vi "Display Tools.vi"(5 "All Default Shortcuts":string[](array[string]), 7 "All Possible Shortcuts":string[](array[string]), 8 "Error In":errorcluster, 10 "Tools":refnum<class "Tools.lvclass">[](array[class]), 11 "Tools Tree Control":refnum<vi>) -> (0 "Error Out":errorcluster, 3 "Shortcuts":map{string, string}(c390))   [LabVIEW 2021, in "Seq Edit Quick Drop.lvlib"]
uses:
  Seq Edit Quick Drop.lvlib
  Dependencies/Tool Menu Utility.lvlibp/Tools/Tools.lvclass
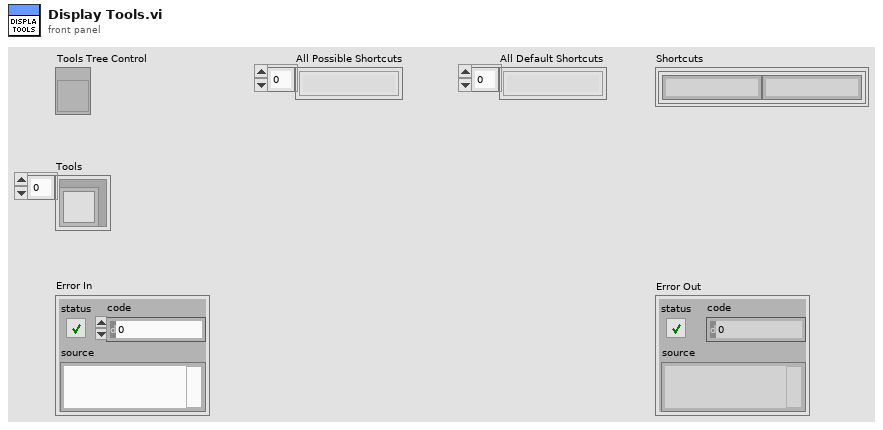
[diagram p1: front panel]
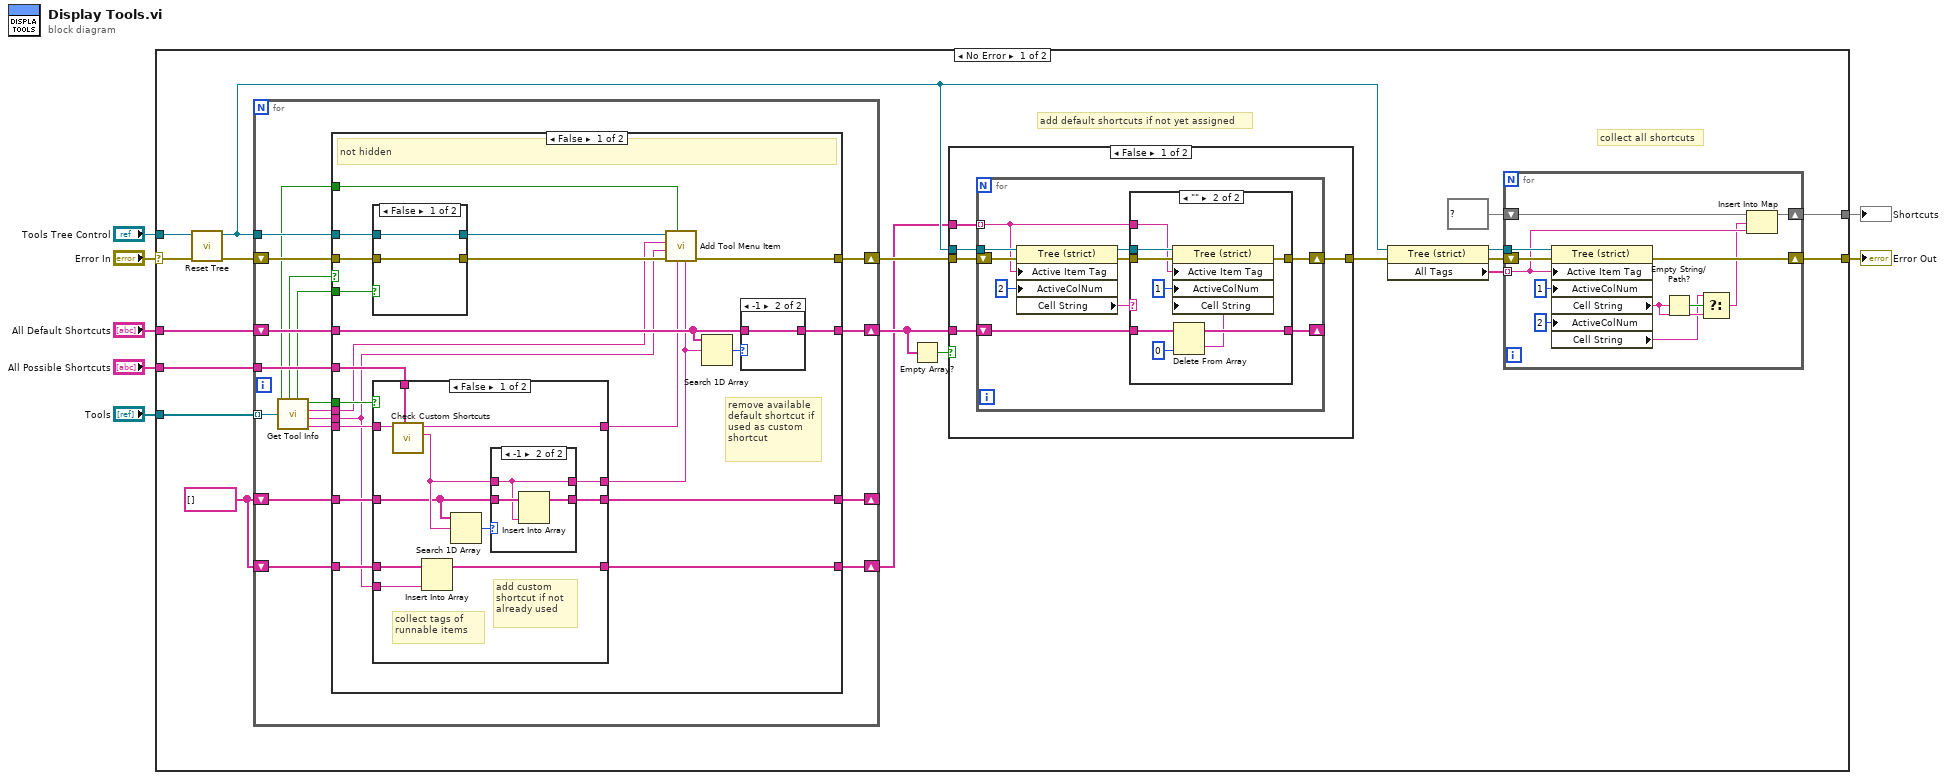
[diagram p0: block diagram]
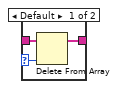
[diagram p4: hidden frame]
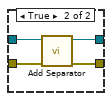
[diagram p5: hidden frame]
diagram:
  n1 = case shown="No Error" "Error In" {
    selector: "Error In" -> [w24 w137]
    tunnel: "Tools" -> [w22 _]
    tunnel: "Tools Tree Control" -> [w25 _]
    tunnel: [w8 w137] -> w4
    tunnel: "All Possible Shortcuts" -> [w23 _]
    tunnel: "All Default Shortcuts" -> [w20 _]
    tunnel: [w13 _] -> w3
    frame No Error {
      w12 = string[] []
      # "collect all shortcuts"
      # "add default shortcuts if not yet assigned"
      n2 = call "Reset Tree.vi"("error in (no error)"=w24, "TreeControl in"=w25) -> ("error out"=w26:errorcluster, "TreeControl out"=w17:refnum<vi>)  [unwired: 8 in]
      n3 = for {
        tunnel: w17 -> [w82]
        shift-right: [w75] -> w21
        shift-left: w26 -> [w83]
        tunnel: w22 -> [w72] mode=indexing
        tunnel: w23 -> [w81]
        shift-right: [w71] -> w19
        shift-left: w20 -> [w80]
        shift-right: [w69] -> _
        shift-left: w12 -> [w70]
        shift-right: [w67] -> w11
        shift-left: w12 -> [w68]
        n4 = call "Get Tool Info.vi"("Tool"=w72) -> ("Enabled?"=w66:bool, "Hidden?"=w74:bool, "Separator Before?"=w73:bool, "Submenu?"=w79:bool, "Parent ID"=w78:string, "ID"=w76:string, "Item Text"=w77:string)  [unwired: 3 in]
        n5 = case shown="False" w74 {
          tunnel: w83 -> [w100 w136]
          tunnel: w82 -> [w99 _]
          tunnel: [w98 w136] -> w75
          tunnel: w73 -> [w97 _]
          tunnel: w79 -> [w95 _]
          tunnel: w78 -> [w89 _]
          tunnel: w77 -> [w96 _]
          tunnel: w76 -> [w84 _]
          tunnel: w81 -> [w92 _]
          tunnel: w80 -> [w102 w135]
          tunnel: [w93 w135] -> w71
          tunnel: w70 -> [w104 w134]
          tunnel: [w103 w134] -> w69
          tunnel: w66 -> [w90 _]
          tunnel: w68 -> [w86 w133]
          tunnel: [w85 w133] -> w67
          frame False {
            # "remove available default shortcut if used as custom shortcut"
            # "not hidden"
            n6 = case shown="False" w97 {
              tunnel: w100 -> [w109 w114]
              tunnel: w99 -> [w110 w113]
              tunnel: [w110 w111] -> w91
              tunnel: [w109 w112] -> w101
              frame False {
              }
              frame True {
                n7 = call "Add Separator.vi"("error in (no error)"=w114, "TreeControl in"=w113) -> ("error out"=w112:errorcluster, "TreeControl out"=w111:refnum<vi>)  [unwired: 8 in]
              }
            }
            n8 = case shown="False" w95 {
              tunnel: w92 -> [w125 _]
              tunnel: w96 -> [w124 w132]
              tunnel: [w123 w132] -> w87
              tunnel: [w121 _] -> w88
              tunnel: w104 -> [w118 w131]
              tunnel: [w120 w131] -> w103
              tunnel: w86 -> [w117 w130]
              tunnel: [w116 w130] -> w85
              tunnel: w84 -> [w115 _]
              frame False {
                # "add custom shortcut if not already used"
                # "collect tags of runnable items"
                n9 = call "Check Custom Shortcuts.vi"("All Possible Shortcuts"=w125, "Item Text"=w124) -> ("Shortcut"=w119:string, "Name"=w123:string)  [unwired: 8 in]
                n10 = Insert Into Array(array=w117, new element=w115) -> (w116:string[])  [unwired: 1 in]
                n11 = Search 1D Array(1D array=w118, element=w119) -> (index of element=w122:i32)  [unwired: 1 in]
                n12 = case shown="-1" w122 {
                  tunnel: [_ w128] -> w121
                  tunnel: w119 -> [_ w128]
                  tunnel: w118 -> [w126 w129]
                  tunnel: [w126 w127] -> w120
                  frame Default {
                  }
                  frame -1 {
                    n13 = Insert Into Array(array=w129, new element=w128) -> (w127:string[])  [unwired: 1 in]
                  }
                }
              }
              frame True {
                # "Submenu"
              }
            }
            n14 = call "Add Tool Menu Item.vi"("Custom Shortcut"=w88, "Name"=w87, "Enabled?"=w90, "Error in"=w101, "ID"=w84, "Parent ID"=w89, "Tools"=w91) -> ("Error Out"=w98:errorcluster)  [unwired: 4 in]
            n15 = Search 1D Array(1D array=w102, element=w88) -> (index of element=w94:i32)  [unwired: 1 in]
            n16 = case shown="-1" w94 {
              selector: w94 -> [w105 _]
              tunnel: [w106 w108] -> w93
              tunnel: w102 -> [w107 w108]
              frame Default {
                n17 = Delete From Array(array=w107, index=w105) -> (array with subset deleted=w106:string[])  [unwired: 1 in, 1 out]
              }
              frame -1 {
              }
            }
          }
          frame True {
            # "hidden"
          }
        }
      }
      n18 = Empty Array?(array=w19) -> (empty?=w18:bool)
      n19 = case shown="False" w18 {
        tunnel: w21 -> [w43 w65]
        tunnel: w17 -> [w42 _]
        tunnel: w11 -> [w41 _]
        tunnel: w19 -> [w40 _]
        tunnel: [w39 w65] -> w9
        frame False {
          n20 = for {
            tunnel: w42 -> [w53]
            shift-right: [w45] -> w39
            shift-left: w43 -> [w52]
            tunnel: w41 -> [w48] mode=indexing
            shift-right: [w46] -> _
            shift-left: w40 -> [w47]
            n21 = property class="Tree (strict)"(reference=w53, error in=w52, "Active Item Tag"=w48, "ActiveColNum"=2 ("Active Cell:Active Column Number")) -> (reference out=w50:refnum<vi>, error out=w49:errorcluster, "Cell String"=w51:string)
            n22 = case shown="\"\"" w51 {
              tunnel: w50 -> [_ w64]
              tunnel: w49 -> [w54 w63]
              tunnel: w48 -> [_ w62]
              tunnel: w47 -> [w55 w60]
              tunnel: [w55 w58] -> w46
              tunnel: [w54 w56] -> w45
              frame Default {
              }
              frame "" {
                n23 = Delete From Array(array=w60, index=0) -> (deleted portion=w57:string, array with subset deleted=w58:string[])  [unwired: 1 in]
                n24 = property class="Tree (strict)"(reference=w64, error in=w63, "Active Item Tag"=w62, "ActiveColNum"=1 ("Active Cell:Active Column Number"), "Cell String"=w57) -> (error out=w56:errorcluster)  [unwired: 1 out]
              }
            }
          }
        }
        frame True {
        }
      }
      n25 = property class="Tree (strict)"(reference=w17, error in=w9) -> (reference out=w15:refnum<vi>, error out=w10:errorcluster, "All Tags"=w16:string[])
      n26 = for {
        tunnel: w16 -> [w28] mode=indexing
        tunnel: w15 -> [w37]
        shift-right: [w32] -> w13
        shift-left: map{string, string} {} ("Size: 0") -> [w31]
        shift-right: [w38] -> w8
        shift-left: w10 -> [w30]
        n27 = property class="Tree (strict)"(reference=w37, error in=w30, "Active Item Tag"=w28, "ActiveColNum"=1 ("Active Cell:Active Column Number"), "ActiveColNum"=2 ("Active Cell:Active Column Number")) -> (error out=w38:errorcluster, "Cell String"=w33:string, "Cell String"=w29:string)  [unwired: 1 out]
        n28 = Empty String/Path?(string/path=w33) -> (empty?=w34:bool)
        n29 = Select(t=w29, s=w34, f=w33) -> (s? t:f=w27:string)
        n30 = Insert Into Map(map in=w31, key=w27, value=w28) -> (map out=w32:map{string, string})  [unwired: 2 out]
      }
    }
    frame Error {
    }
  }
  "Error Out" <- w4
  "Shortcuts" <- w3
